vi "Set DDS Pinlv.vi"(8 "error in (no error)":errorcluster, 10 "pinlv":u32, 11 "channel_index":u8) -> (0 "error out":errorcluster)   [LabVIEW 2021, in "vmmso.lvlib"]
doc: "DLL_API void WINAPI SetDDSPinlv(unsigned char channel_index, unsigned int pinlv);"
uses:
  vmmso.lvlib
  vmmso.dll
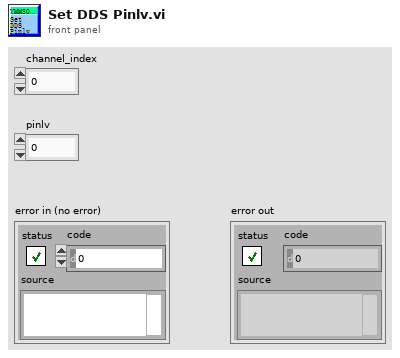
[diagram p1: front panel]
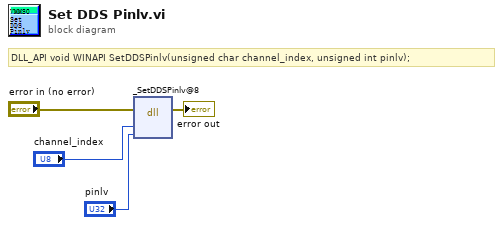
[diagram p0: block diagram]
diagram:
  # "DLL_API void WINAPI SetDDSPinlv(unsigned char channel_index, unsigned int pinlv);"
  n1 = dll-call lib="O:/MSO/library/demo-Labview/vmmso/vmmso.*" fn="_SetDDSPinlv@8"(error in="error in (no error)", "channel_index"="channel_index", "pinlv"="pinlv") -> (error out=→"error out":errorcluster)  [unwired: 5 in, 1 out]
